vi "Extract Server Command Specifier.vi"(11 "Data":u8[](array[numeric])) -> (3 "Server Command Specifier":u8)   [LabVIEW 2020, in "CANopen.lvlib" / "SDO Manager.lvlib" / "SDO Transfer.lvclass"]
uses:
  SDO Transfer.lvclass
  SDO Transfer.lvclass/SDO Transfer.ctl
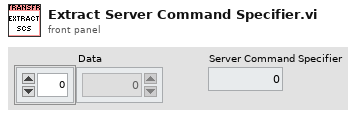
[diagram p1: front panel]
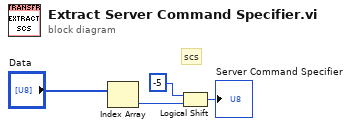
[diagram p0: block diagram]
diagram:
  # "scs"
  n1 = Index Array(array="Data") -> (element=w3:u8)  [unwired: 1 in]
  n2 = Logical Shift(y=i16 -5, x=w3) -> (x << y=→"Server Command Specifier":u8)
